vi "Initiate.vi"(8 "error in":errorcluster, 10 "configuration":T1, 11 "session in":T2) -> (0 "error out":errorcluster)   [LabVIEW 2021, in "dcvmDPI_AD7606B_serverImpl.lvlib"]
uses:
  dcvmDPI_AD7606B_serverImpl.lvlib
  controls/session.ctl
  controls/configuration.ctl
  <instrlib>/niDigital/niDigital.llb/niDigital Burst Pattern (Burst Only).vi
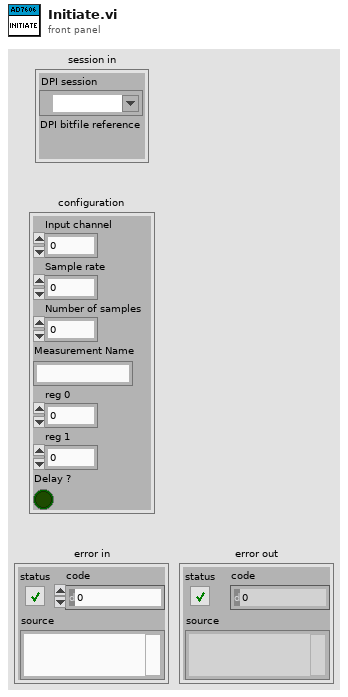
[diagram p1: front panel]
types:
  T1 = typedef "dcvmDPI_AD7606B_serverImpl.lvlib/configuration.ctl" = cluster{"Input channel":i32, "Sample rate":dbl, "Number of samples":u32, "Measurement Name":string, "reg 0":i32, "reg 1":i32, "Delay ?":bool}
  T2 = typedef "dcvmDPI_AD7606B_serverImpl.lvlib/session.ctl" = cluster{"DPI session":refnum<k15>, "DPI bitfile reference":refnum<k20>}
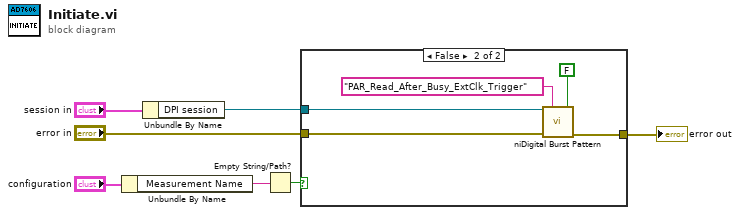
[diagram p0: block diagram]
diagram:
  n1 = Unbundle By Name("configuration") -> ("Measurement Name"=w2:string)
  n2 = Unbundle By Name("session in") -> ("DPI session"=w4:refnum<k15>)
  n3 = Empty String/Path?(string/path=w2) -> (empty?=w1:bool)
  n4 = case shown="False" w1 {
    tunnel: [w8 w12] -> w7
    tunnel: "error in" -> [w8 w9]
    tunnel: w4 -> [_ w10]
    frame True {
    }
    frame False {
      n5 = call-poly <instrlib>:"niDigital Burst Pattern.vi"("instrument handle"=w10, "start label"="PAR_Read_After_Busy_ExtClk_Trigger", "wait until done? (T)"=FALSE, "error in"=w9) -> ("error out"=w12:errorcluster)  [unwired: 10 in, 1 out]
    }
  }
  "error out" <- w7
